vi "SLL DE DO Safe Values.vi"(8 "error in (no error)":errorcluster) -> (0 "error out":errorcluster, 2 "DO Safe Values":bool[](array[boolean]), 3 "DO Name":T1[](array[typedef]))   [LabVIEW 2013]
doc: "Copyright © 2005, Soliton Technologies.\nAll rights reserved."
uses:
  Controls/SLL DE List of Digital Outputs.ctl
  Controls/SLL DE DO Safe Value Global Options.ctl
panel:
  in  "List of Digital Outputs":T1=enum."STATION1_STOP TEST"
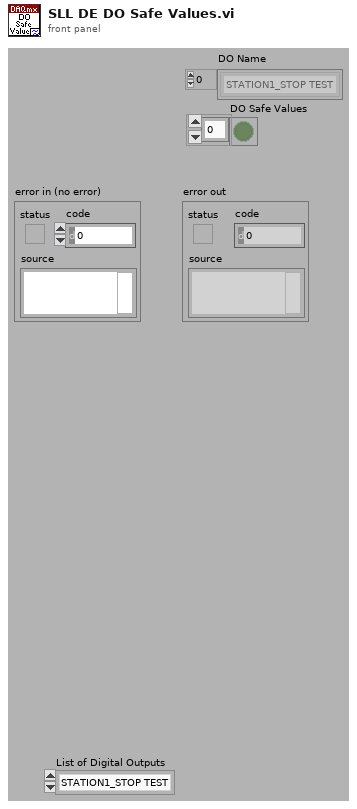
[diagram p1: front panel]
types:
  T1 = typedef "SLL DE List of Digital Outputs.ctl" = enum16{"STATION1_START TEST", "STATION1_STOP TEST", "STATION1_LIGHT1", "STATION1_LIGHT2", "STATION1_LIGHT3", "STATION1_SELECT_TEST", "STATION2_START TEST", "STATION2_STOP TEST", "STATION2_LIGHT1", "STATION2_LIGHT2", "STATION2_LIGHT3", "STATION2_SELECT_TEST", "STATION3_START TEST", "STATION3_STOP TEST", "STATION3_LIGHT1", "STATION3_LIGHT2", "STATION3_LIGHT3", "STATION3_SELECT_TEST", "STATION4_START TEST", "STATION4_STOP TEST", "STATION4_LIGHT1", "STATION4_LIGHT2", "STATION4_LIGHT3", "STATION4_SELECT_TEST"}
  T2 = typedef "SLL DE DO Safe Value Global Options.ctl" = enum16{"Read", "Write"}
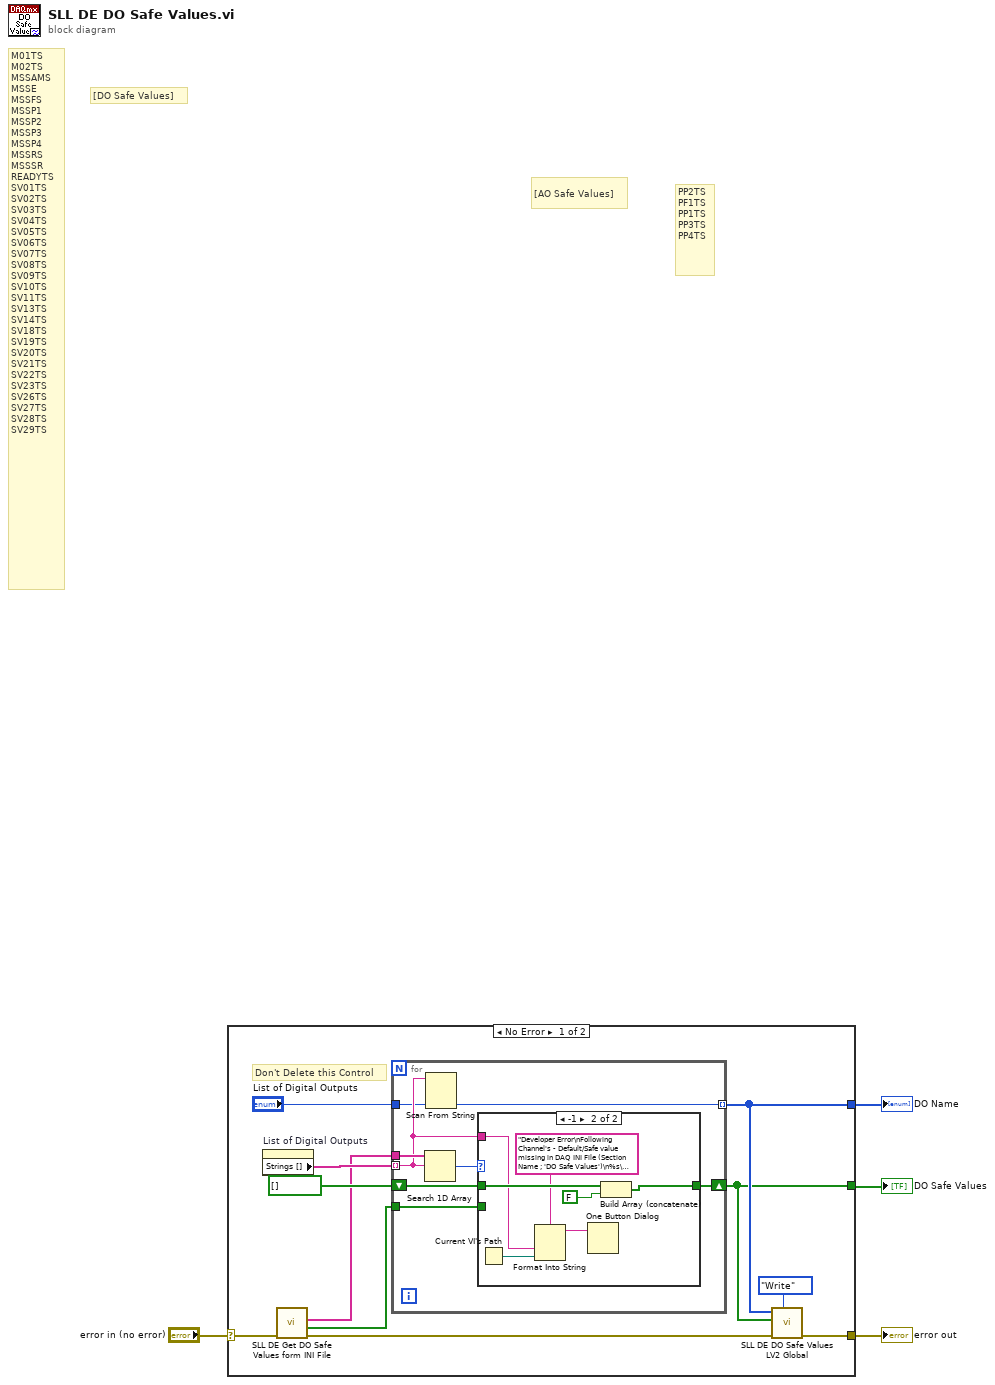
[diagram p0: block diagram]
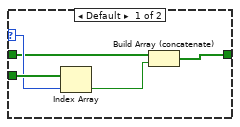
[diagram p2: hidden frame]
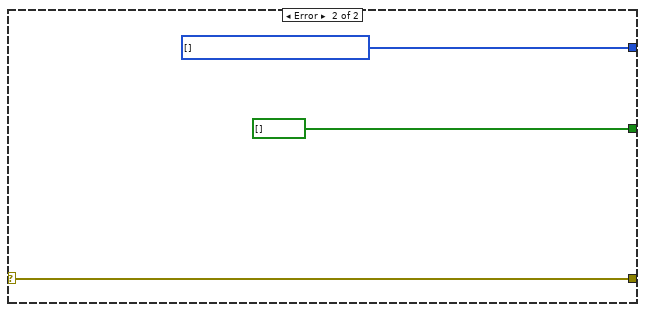
[diagram p3: hidden frame]
diagram:
  # "[DO Safe Values]"
  # "PP2TS\nPF1TS\nPP1TS\nPP3TS\nPP4TS"
  # "[AO Safe Values]"
  # "M01TS\nM02TS\nMSSAMS\nMSSE\nMSSFS\nMSSP1\nMSSP2\nMSSP3\nMSSP4\nMSSRS\nMSSSR\nREADYTS\nSV01TS\nSV02TS\nSV03TS\nSV04TS\nSV05TS\nSV06TS\nSV07TS\nSV08TS\nSV09TS\nSV10TS\nSV11TS\nSV13TS\nSV14TS\nSV18TS\nSV19TS\nSV20TS\nSV21TS\nSV22TS\nSV23TS\nSV26TS\nSV27TS\nSV28TS\nSV29TS"
  n1 = case shown="No Error" "error in (no error)" {
    selector: "error in (no error)" -> [w8 w38]
    tunnel: [w11 w38] -> w3
    tunnel: [w9 bool[] [] ("Key Values")] -> w2
    tunnel: [w10 w36] -> w1
    frame No Error {
      # "Don't Delete this Control"
      n2 = property on="List of Digital Outputs" class="Enum (strict)"() -> ("Strings []"=w15:string[])  [unwired: 2 in, 2 out]
      n3 = call "SLL DE Get DO Safe Values form INI File.vi"("error in (no error)"=w8) -> ("error out"=w7:errorcluster, "DO Safe Values"=w6:bool[], "DO Channel Names (String)"=w5:string[])  [unwired: 7 in, 1 out]
      n4 = for {
        tunnel: w5 -> [w23]
        tunnel: w15 -> [w18] mode=indexing
        tunnel: w6 -> [w21]
        shift-right: [w20] -> w9
        shift-left: bool[] [] -> [w19]
        tunnel: "List of Digital Outputs" -> [w17]
        tunnel: [w16] -> w10 mode=indexing
        n5 = Search 1D Array(1D array=w23, element=w18) -> (index of element=w22:i32)  [unwired: 1 in]
        n6 = Scan From String(input string=w18, default 1=w17) -> (output 1=w16:T1)  [unwired: 3 in, 3 out]
        n7 = case shown="-1" w22 {
          selector: w22 -> [w27 _]
          tunnel: w21 -> [w28 _]
          tunnel: [w26 w33] -> w20
          tunnel: w19 -> [w24 w35]
          tunnel: w18 -> [_ w29]
          frame Default {
            n8 = Index Array(array=w28, index=w27) -> (element=w25:bool)
            n9 = Build Array (concatenate)(w24, w25) -> (w26:bool[])
          }
          frame -1 {
            n10 = Current VI's Path() -> (path=w32:path)
            n11 = Format Into String(format string="Developer Error\nFollowing Channel's - Default/Safe value missing in DAQ INI File (Section Name ; 'DO Safe Values')\n%s\n%s" ("message"), w29, w32) -> (resulting string=w31:string)  [unwired: 2 in, 1 out]
            n12 = One Button Dialog(message=w31) -> ()  [unwired: 1 in, 1 out]
            n13 = Build Array (concatenate)(w35, FALSE) -> (w33:bool[])
          }
        }
      }
      n14 = call "SLL DE DO Safe Values LV2 Global.vi"("Cases"=SLL_DE_DO_Safe_Value_Global_Options."Write", "error in (no error)"=w7, "Value In"=w9, "Elements In"=w10) -> ("error out"=w11:errorcluster)  [unwired: 5 in, 2 out]
    }
    frame Error {
      w36 = T1[] [] items=["STATION1_START TEST", "STATION1_STOP TEST", "STATION1_LIGHT1", "STATION1_LIGHT2", "STATION1_LIGHT3", "STATION1_SELECT_TEST", "STATION2_START TEST", "STATION2_STOP TEST", "STATION2_LIGHT1", "STATION2_LIGHT2", "STATION2_LIGHT3", "STATION2_SELECT_TEST", "STATION3_START TEST", "STATION3_STOP TEST", "STATION3_LIGHT1", "STATION3_LIGHT2", "STATION3_LIGHT3", "STATION3_SELECT_TEST", "STATION4_START TEST", "STATION4_STOP TEST", "STATION4_LIGHT1", "STATION4_LIGHT2", "STATION4_LIGHT3", "STATION4_SELECT_TEST"]
    }
  }
  "error out" <- w3
  "DO Name" <- w1
  "DO Safe Values" <- w2
